vi "Function FGV.vi"(7 "Enum 3":T1, 8 "error constant":errorcluster, 10 "Enum in":enum16{"Check account", "Withdraw", "Deposit"}(ring)) -> (0 "error IO":errorcluster, 2 "Enum out":enum16{"Check account", "Withdraw", "Deposit"}(ring))   [LabVIEW 2013]
uses:
  Function states.ctl
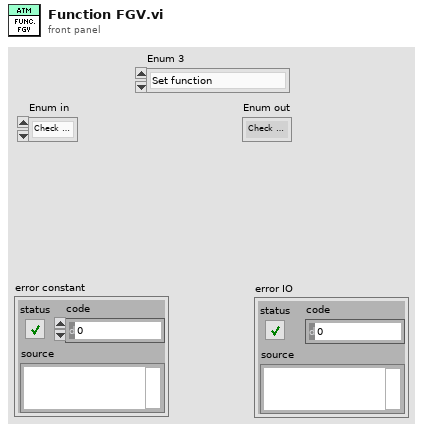
[diagram p1: front panel]
types:
  T1 = typedef "Function states.ctl" = enum16{"Set function", "Get function"}
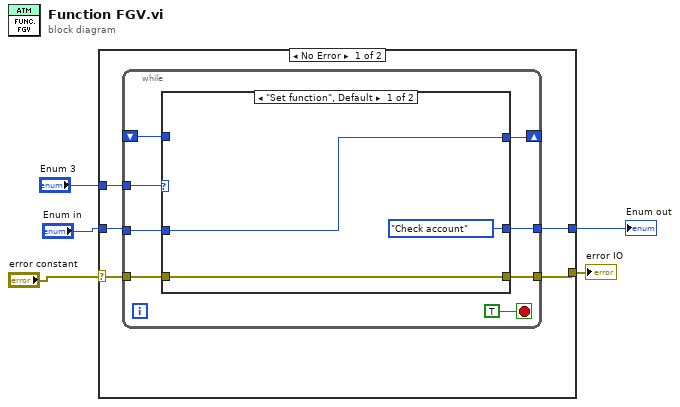
[diagram p0: block diagram]
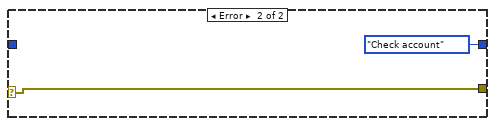
[diagram p3: hidden frame]
diagram:
  n1 = case shown="No Error" "error constant" {
    selector: "error constant" -> [w6 w25]
    tunnel: [w10 enum16{"Check account", "Withdraw", "Deposit"}."Check account" ("Enum in")] -> w5
    tunnel: "Enum in" -> [w9 _]
    tunnel: "Enum 3" -> [w8 _]
    tunnel: [w7 w25] -> w1
    frame No Error {
      n2 = while {
        tunnel: w8 -> [w17]
        tunnel: w9 -> [w16]
        shift-right: [w15] -> _
        shift-left: _ -> [w14]
        tunnel: [w13] -> w10
        tunnel: [w12] -> w7
        tunnel: w6 -> [w11]
        stop <- TRUE stop-if-true
        n3 = case shown="\"Set function\", Default" w17 {
          tunnel: w16 -> [w21 _]
          tunnel: [w21 w23] -> w15
          tunnel: w14 -> [_ w23]
          tunnel: [enum16{"Check account", "Withdraw", "Deposit"}."Check account" ("Enum in") w23] -> w13
          tunnel: [w19 w22] -> w12
          tunnel: w11 -> [w19 w22]
          frame "Set function", Default {
          }
          frame "Get function" {
          }
        }
      }
    }
    frame Error {
    }
  }
  "Enum out" <- w5
  "error IO" <- w1
